vi "Lab Arreglos-4.vi"() -> ()   [LabVIEW 2018]
panel:
  out "Array":void[](array[numeric])
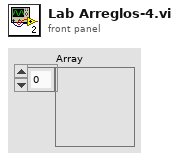
[diagram p1: front panel]
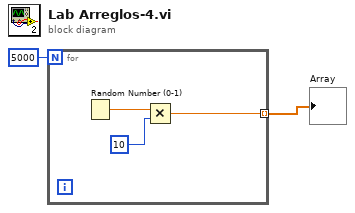
[diagram p0: block diagram]
diagram:
  n1 = for {
    N: 5000 -> [_]
    tunnel: [w4] -> w1 mode=indexing
    n2 = Random Number (0-1)() -> (number: 0 to 1=w5:dbl)
    n3 = Multiply(x=w5, y=10) -> (x*y=w4:dbl)
  }
  "Array" <- w1
